vi "Is This Control Of This LabVIEW Class.vi"(8 "error in (no error)":errorcluster, 10 "LVClass Refnum":refnum<vi>, 11 "Ctl Refnum":refnum<vi>) -> (0 "error out":errorcluster, 1 "Is this control of this class?":bool, 2 "LVClass Refnum out":refnum<vi>, 3 "Ctl Refnum out":refnum<vi>)   [LabVIEW 2020]
doc: "Given a control refnum and a LVClass refnum, this VI determines whether the control is a control of the LVClass type. The VI will return true for the LVClass' regular class controls/indicators and for XControls whose type is the given LVClass. \n\nThis VI will return a \"not supported\" error in built applications."
uses:
  <vilib>/Utility/Data Type/NI_Data Type.lvlib
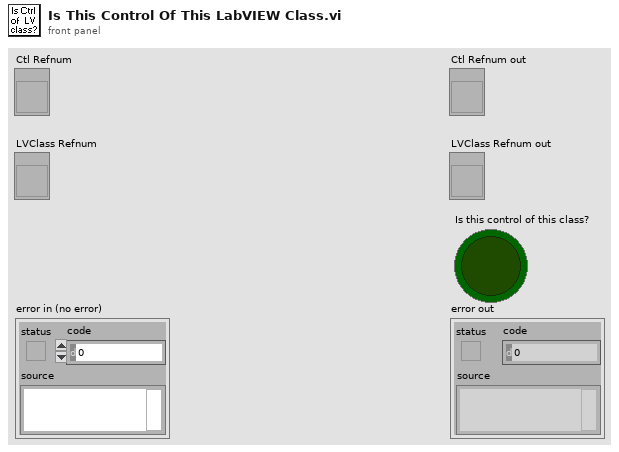
[diagram p1: front panel]
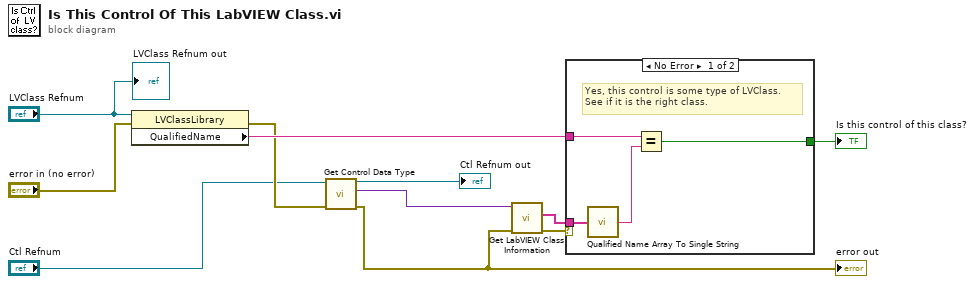
[diagram p0: block diagram]
diagram:
  n1 = property class="LVClassLibrary"(reference="LVClass Refnum", error in="error in (no error)") -> (error out=w6:errorcluster, "QualifiedName"=w7:string)  [unwired: 1 out]
  n2 = call <vilib>:"Get Control Data Type.vi"("error in (no error)"=w6, "Control Refnum in"="Ctl Refnum") -> ("error out"=w3:errorcluster, "Control's Data Type"=w10:variant, "Control Refnum out"=→"Ctl Refnum out":refnum<vi>)  [unwired: 3 in]
  "error out" <- w3
  n3 = call <vilib>:"Get LabVIEW Class Information.vi"("error in (no error)"=w3, "variant"=w10) -> ("error out"=w8:errorcluster, "qualified LabVIEW class name"=w9:string[])  [unwired: 7 in, 1 out]
  n4 = case shown="No Error" w8 {
    tunnel: w9 -> [w15 _]
    tunnel: [w12 _] -> w11
    tunnel: w7 -> [w13 _]
    frame No Error {
      # "Yes, this control is some type of LVClass. \nSee if it is the right class."
      n5 = call <vilib>:"Qualified Name Array To Single String.vi"("Fully Qualified Array"=w15) -> ("Fully Qualified String"=w14:string)
      n6 = Equal?(x=w13, y=w14) -> (x = y?=w12:bool)
    }
    frame Error {
      # "Don't propagate this error. An error generated here just means the control is not an LVClass control."
    }
  }
  "Is this control of this class?" <- w11
  "LVClass Refnum out" <- "LVClass Refnum"
